vi "DISPlay_LABel.vi"(7 "Write?":bool, 8 "Error":errorcluster caption="错误输入（无错误）", 10 "Channel":u32, 11 "VISA resource name":refnum<visa-resource-name>) -> (0 "Error out":errorcluster, 2 "Channel out":u32, 3 "VISA resource name out":refnum<visa-resource-name>)   [LabVIEW 2020]
doc: "通道标签"
panel:
  out "读取缓冲区":string
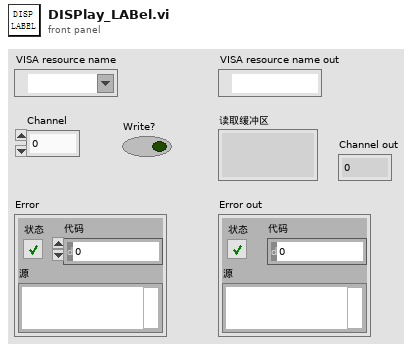
[diagram p1: front panel]
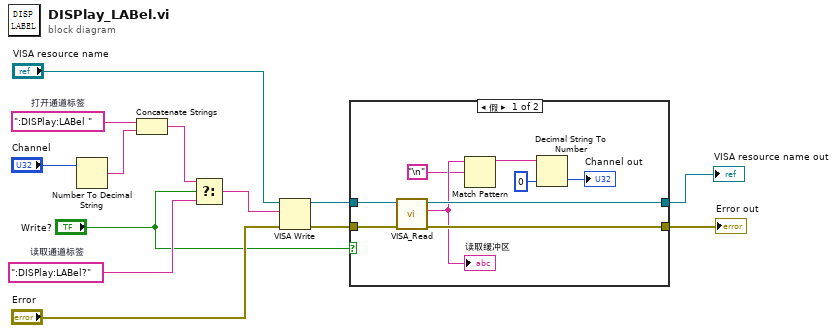
[diagram p0: block diagram]
diagram:
  w8 = ":DISPlay:LABel?"  # 读取通道标签
  w12 = ":DISPlay:LABel "  # 打开通道标签
  n1 = Number To Decimal String(number="Channel") -> (decimal integer string=w11:string)  [unwired: 1 in]
  n2 = Concatenate Strings(w12, w11) -> (w9:string)
  n3 = Select(t=w9, s="Write?", f=w8) -> (s? t:f=w7:string)
  n4 = VISA Write(VISA resource name="VISA resource name", write buffer=w7, error in (no error)="Error") -> (VISA resource name out=w3:refnum<visa-resource-name>, error out=w5:errorcluster)  [unwired: 1 out]
  n5 = case shown="假" "Write?" {
    tunnel: w3 -> [w22 w24]
    tunnel: w5 -> [w21 w23]
    tunnel: [w19 w23] -> w4
    tunnel: [w20 w24] -> w1
    frame False {
      n6 = call "VISA_Read.vi"("Error"=w21, "VISA resource name"=w22) -> ("Error out"=w19:errorcluster, "读取缓冲区"=w18:string, "VISA resource name out"=w20:refnum<visa-resource-name>)  [unwired: 7 in]
      "读取缓冲区" <- w18
      n7 = Match Pattern(string=w18, regular expression="\n") -> (before substring=w15:string)  [unwired: 1 in, 3 out]
      n8 = Decimal String To Number(string=w15, default (0L)=u32 0 ("默认(0 I32)")) -> (number=→"Channel out":u32)  [unwired: 1 in, 1 out]
    }
    frame True {
    }
  }
  "VISA resource name out" <- w1
  "Error out" <- w4
